vi "Parse drawing operation.vi"(0 "picture data in":string, 4 "offset":i32, 7 "picture size":u32) -> (13 "last element":bool, 14 "picture data out":string, 15 "op-code":T1 items=["set pixel"=4, "move pen"=5, "move pen to"=6, "draw line"=7, "draw line to"=8, "rectangle frame"=9, "rectangle fill"=10, "oval frame"=11, "oval fill"=12, "arc frame"=13, "arc fill"=14, "gray out rect"=15, "poly line"=16, "poly line fill"=17, "text box"=18, "round rect frame"=24, "round rect fill"=25, "copy pixmap"=29, "new font"=0, "copy pixmap with mask"=40, "select pen"=41], 16 "data length":u32, 17 "data string":string, 18 "offset past element":i32)   [LabVIEW 2016, in "LV Object Event Registration Node.xnode"]
uses:
  LV Object Event Registration Node.xnode
  picture op-code.ctl
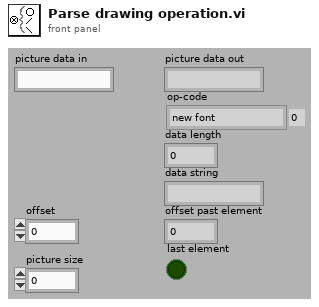
[diagram p1: front panel]
types:
  T1 = typedef "LV Object Event Registration Node.xnode/picture op-code.ctl" = u16
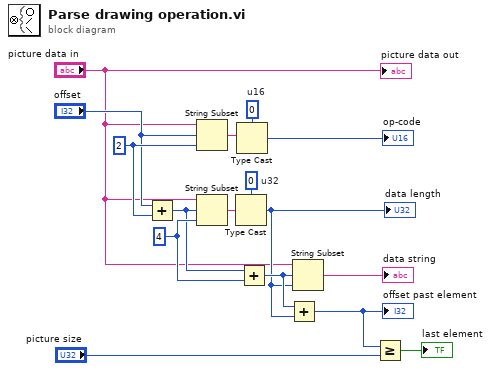
[diagram p0: block diagram]
diagram:
  w12 = u32 0  # u32
  w15 = 4 ("length (rest)")
  w7 = u16 0  # u16
  w11 = 2 ("length (rest)")
  n1 = Add(x="offset", y=w11) -> (x+y=w14:i32)
  n2 = String Subset(string="picture data in", offset (0)="offset", length (rest)=w11) -> (substring=w8:string)
  n3 = String Subset(string="picture data in", offset (0)=w14, length (rest)=w15) -> (substring=w13:string)
  n4 = Type Cast(type=w12, x=w13) -> (*(type *) &x=w5:u32)
  "data length" <- w5
  n5 = Type Cast(type=w7, x=w8) -> (*(type *) &x=→"op-code":u16)
  n6 = Add(x=w14, y=w15) -> (x+y=w6:i32)
  n7 = Add(x=w6, y=w5) -> (x+y=w3:u32)
  "offset past element" <- w3
  n8 = String Subset(string="picture data in", offset (0)=w6, length (rest)=w5) -> (substring=→"data string":string)
  n9 = Greater Or Equal?(x=w3, y="picture size") -> (x >= y?=→"last element":bool)
  "picture data out" <- "picture data in"
